vi "Get Environment.vi"(8 "error in":errorcluster, 11 "Paths":T1) -> (0 "error out":errorcluster, 3 "Environment out":refnum<k24>)   [LabVIEW 2020, in "WebView2 Control.xctl"]
uses:
  WebView2 Control.xctl
  E:/Labview/LV 2020/Libs/LV-WebView2/microsoft.web.webview2/lib/net45/Microsoft.Web.WebView2.Core.dll
  microsoft.web.webview2/lib/net45/Microsoft.Web.WebView2.Core.dll
  Paths.ctl
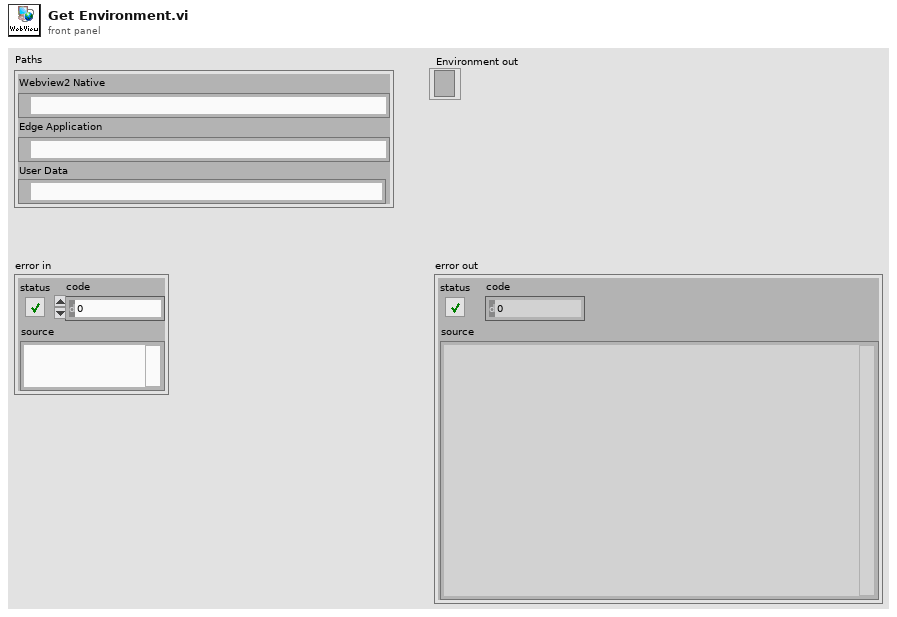
[diagram p1: front panel]
types:
  T1 = typedef "WebView2 Control.xctl/Paths.ctl" = cluster{"Webview2 Native":path, "Edge Application":path, "User Data":path}
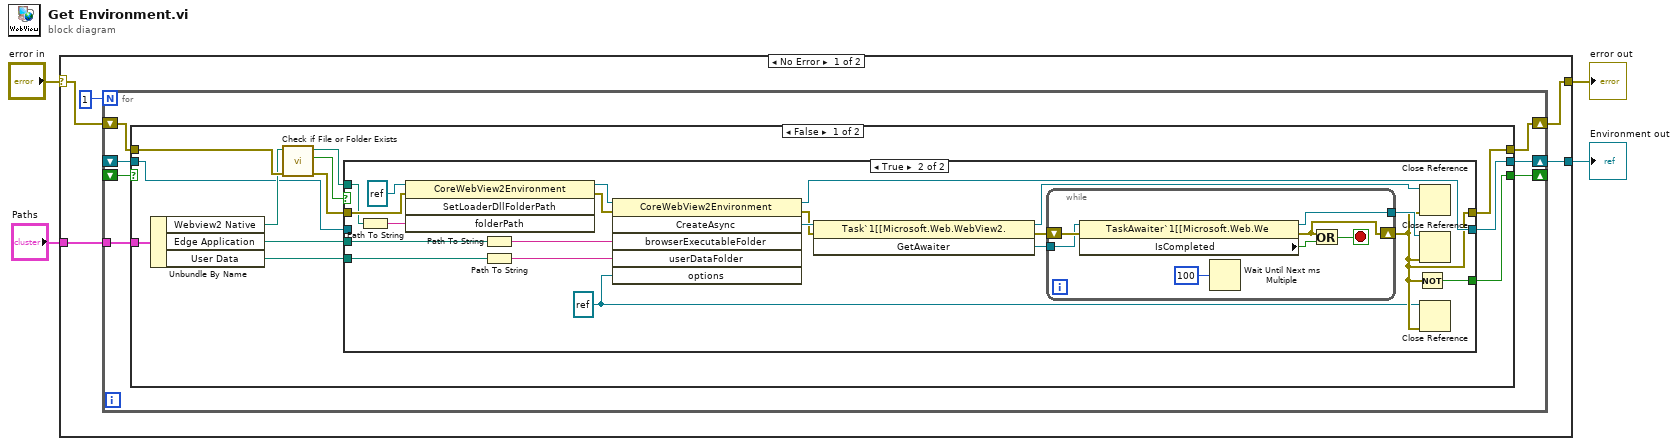
[diagram p0: block diagram]
diagram:
  n1 = case shown="No Error" "error in" {
    selector: "error in" -> [w6 w61]
    tunnel: [w9 w61] -> w4
    tunnel: [w8 _] -> w3
    tunnel: "Paths" -> [w7 _]
    frame No Error {
      n2 = for {
        N: 1 -> [_]
        tunnel: w7 -> [w16]
        shift-right: [w14] -> w8
        shift-left: _ -> [w13]
        shift-right: [w15] -> w9
        shift-left: w6 -> [w12]
        shift-right: [w11] -> _
        shift-left: _ -> [w10]
        n3 = case shown="False" w10 {
          selector: w10 -> [_ w58]
          tunnel: w16 -> [w26 _]
          tunnel: [w23 w59] -> w15
          tunnel: [w25 w60] -> w14
          tunnel: w13 -> [w17 w60]
          tunnel: w12 -> [w24 w59]
          tunnel: [w22 w58] -> w11
          frame False {
            n4 = Unbundle By Name(w26) -> ("Webview2 Native"=w20:path, "Edge Application"=w28:path, "User Data"=w27:path)
            n5 = call <vilib>:"Check if File or Folder Exists.vi"("error in (no error)"=w24, "path"=w20) -> ("error out"=w21:errorcluster, "file or folder exists?"=w18:bool, "dup path"=w19:path)  [unwired: 7 in]
            n6 = case shown="True" w18 {
              tunnel: w28 -> [_ w43]
              tunnel: w27 -> [_ w42]
              tunnel: [w30 w36] -> w25
              tunnel: [w29 w35] -> w23
              tunnel: [_ w34] -> w22
              tunnel: w21 -> [w29 w32]
              tunnel: w19 -> [_ w31]
              tunnel: w17 -> [w30 _]
              frame False {
              }
              frame True {
                w33 = refnum<k24> refnum ("options")
                n7 = Path To String(path=w31) -> (string=w46:string)
                n8 = invoke class="CoreWebView2Environment" method="SetLoaderDllFolderPath"(reference=refnum<k24> refnum ("environment"), error in=w32, "folderPath"=w46) -> (reference out=w49:refnum<k24>, error out=w48:errorcluster)  [unwired: 1 in, 2 out]
                n9 = Path To String(path=w43) -> (string=w45:string)
                n10 = Path To String(path=w42) -> (string=w47:string)
                n11 = invoke class="CoreWebView2Environment" method="CreateAsync"(reference=w49, error in=w48, "browserExecutableFolder"=w45, "userDataFolder"=w47, "options"=w33) -> (reference out=w36:refnum<k24>, error out=w38:errorcluster, "CreateAsync"=w44:refnum<k24>)  [unwired: 1 in, 3 out]
                n12 = invoke class="Task`1[[Microsoft.Web.WebView2." method="GetAwaiter"(reference=w44, error in=w38) -> (reference out=w37:refnum<k24>, error out=w40:errorcluster, "GetAwaiter"=w41:refnum<k24>)  [unwired: 1 in]
                n13 = while {
                  tunnel: w41 -> [w56]
                  shift-right: [w51] -> w35
                  shift-left: w40 -> [w57]
                  tunnel: [w53] -> w39
                  stop <- w52 stop-if-true
                  n14 = property class="TaskAwaiter`1[[Microsoft.Web.We"(reference=w56, error in=w57) -> (reference out=w53:refnum<k24>, error out=w51:errorcluster, "IsCompleted"=w54:bool)
                  n15 = Wait Until Next ms Multiple(millisecond multiple=u32 100) -> ()  [unwired: 1 out]
                  n16 = Or(x=w51, y=w54) -> (x .or. y?=w52:bool)
                }
                n17 = Not(x=w35) -> (.not. x?=w34:bool)
                n18 = Close Reference(reference=w37, error in (no error)=w35) -> ()  [unwired: 1 out]
                n19 = Close Reference(reference=w39, error in (no error)=w35) -> ()  [unwired: 1 out]
                n20 = Close Reference(reference=w33, error in (no error)=w35) -> ()  [unwired: 1 out]
              }
            }
          }
          frame True {
          }
        }
      }
    }
    frame Error {
    }
  }
  "error out" <- w4
  "Environment out" <- w3
